vi "Read_Camera.vi"(0 "Camera":T2, 1 "node":string, 3 "error in":errorcluster) -> (2 "ROS Image":T1, 4 "Reply":string, 5 "image out":T3 {"Dialogs" format="%.0b"}, 6 "picture":picture, 7 "error out":errorcluster)   [LabVIEW 2013]
doc: "Get an image from one of Baxter's hand cameras. \n\nIt is highly recommended that you are connected to baxter via ethernet rather than over wireless when doing this."
uses:
  ROS/Code/SubVIs/BaxterCamera.ctl
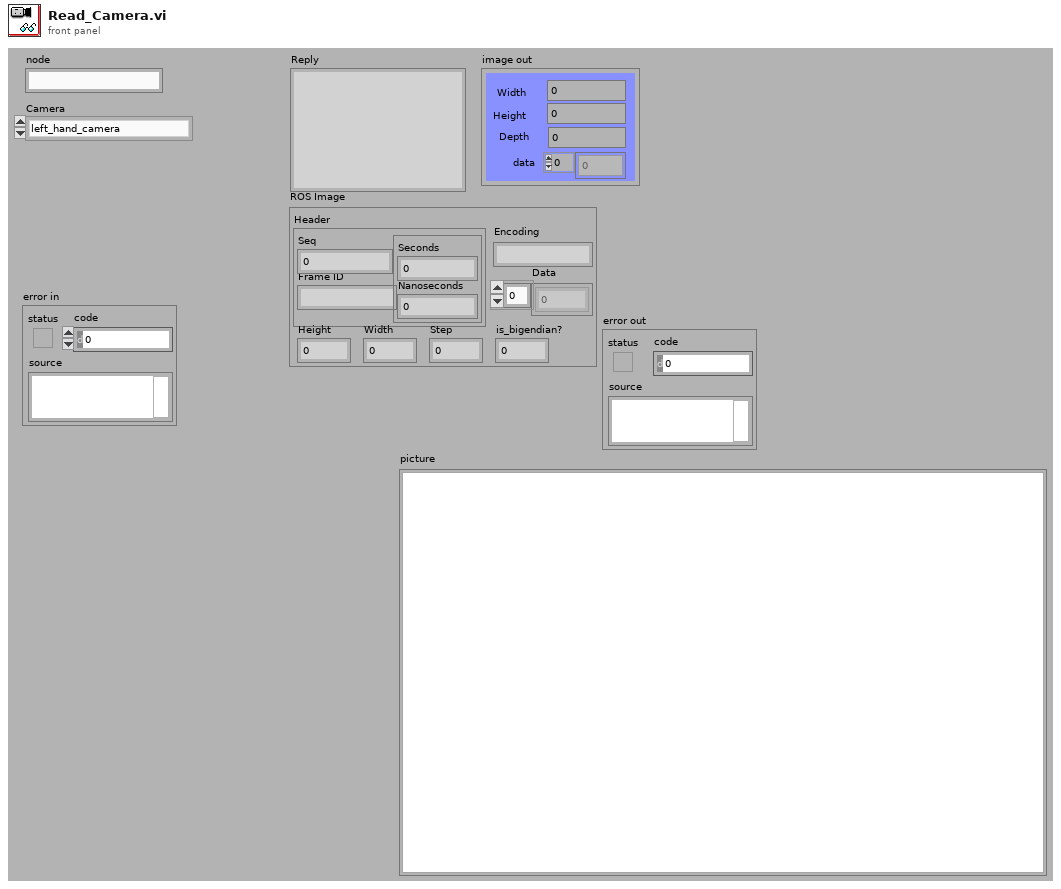
[diagram p1: front panel]
types:
  T1 = cluster{"Header":cluster{"Seq":u32, "Frame ID":string, cluster{"Seconds":i32, "Nanoseconds":i32}}, "Height":u32, "Width":u32, "is_bigendian?":u8, "Step":u32, "Data":u8[], "Encoding":string}
  T2 = typedef "BaxterCamera.ctl" = enum16{"left_hand_camera", "right_hand_camera", "head_camera"}
  T3 = cluster{"Width":i32, "Height":i32, "Depth":i32, "data":u8[], "Compressed data":u8[], "Color table":u32[], "Duration":i32, "Options":i32, "Timestamp":i32, "ID":i32, "Reserved":i32, "Dialogs":u32}
  T4 = typedef "_ROSControl.ctl" = cluster{"topic port":u16, "Node":string, "topic":string, "type":string, "node port":u32, "error ":errorcluster, "Direction":T5, "APIs":string[]}
  T5 = typedef "_ROSDirection.ctl" = enum16{"Node", "Publisher", "Subscriber", "Service Client"}
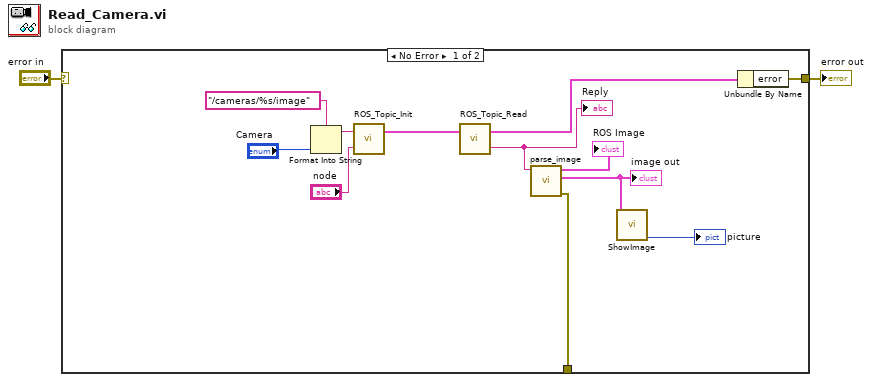
[diagram p0: block diagram]
diagram:
  n1 = case shown="No Error" "error in" {
    selector: "error in" -> [_ w15]
    tunnel: [w14 w15] -> w2
    tunnel: [w7 _] -> _
    frame No Error {
      n2 = Format Into String(format string="/cameras/%s/image" ("topic"), "Camera") -> (resulting string=w9:string)  [unwired: 2 in, 1 out]
      n3 = call "ROS_Topic_Init.vi"("node"="node", "topic"=w9) -> ("ROS out"=w12:T4)  [unwired: 1 in]
      n4 = call "ROS_Topic_Read.vi"("ROS in"=w12) -> ("Reply"=w8:string, "ROS out"=w11:T4)  [unwired: 1 in]
      "Reply" <- w8
      n5 = call "parse_image.vi"("msg in"=w8) -> ("ROS Image"=→"ROS Image":T1, "Image Out"=w4:T3, "error out"=w7:errorcluster)  [unwired: 5 in, 1 out]
      "image out" <- w4
      n6 = call "ShowImage.vi"("Image"=w4) -> ("picture"=→"picture":picture)  [unwired: 10 in]
      n7 = Unbundle By Name(w11) -> ("error"=w14:errorcluster)
    }
    frame Error {
    }
  }
  "error out" <- w2
